vi "WinCI Add From SCC.vi"(8 "error in":errorcluster, 10 "files":path[](array[path]), 11 "source control reference in":T1) -> (0 "error out":errorcluster, 2 "status message":string, 3 "source control reference out":T1)   [LabVIEW 2017, in "NI_SCC_WinCI.lvlib"]
uses:
  <vilib>/SourceControl/Providers/WinCI/NI_SCC_WinCI.lvlib
  <vilib>/SourceControl/sccapi/SCCAPI Refnum.ctl
  <vilib>/SourceControl/sccapi/NI_SCC.lvlib
panel:
  out "result":i32
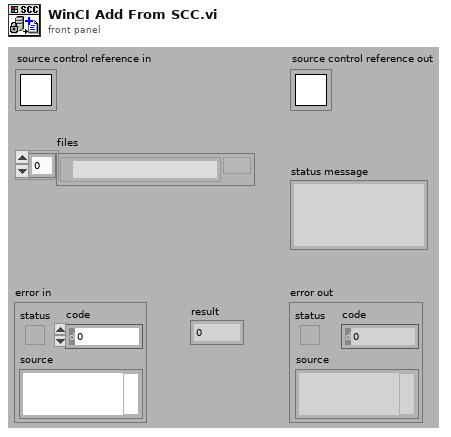
[diagram p1: front panel]
types:
  T1 = typedef "NI_SCC.lvlib/SCCAPI Refnum.ctl" = refnum<k1>
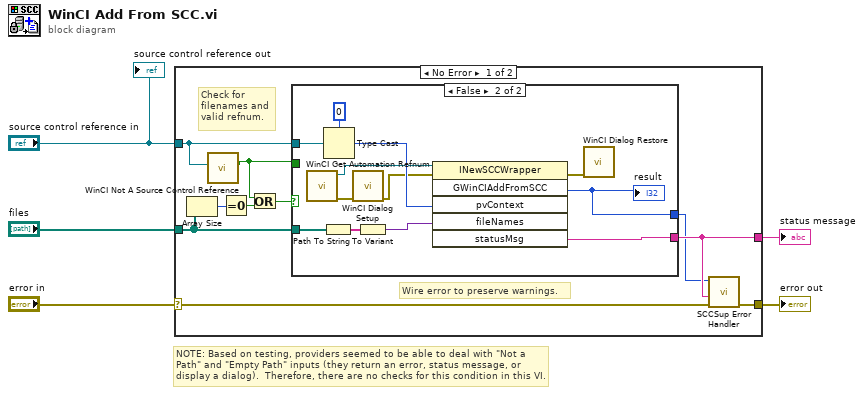
[diagram p0: block diagram]
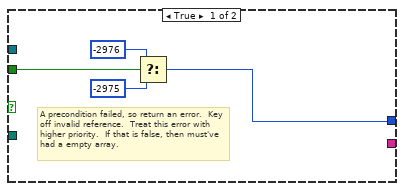
[diagram p2: hidden frame]
diagram:
  # "NOTE: Based on testing, providers seemed to be able to deal with \"Not a Path\" and \"Empty Path\" inputs (they return an error, status message, or display a dialog).  Therefore, there are no checks for this condition in this VI."
  n1 = case shown="No Error" "error in" {
    selector: "error in" -> [w8 w32]
    tunnel: [w14 w32] -> w4
    tunnel: "source control reference in" -> [w7 _]
    tunnel: [w13 _] -> w2
    tunnel: "files" -> [w15 _]
    frame No Error {
      # "Check for filenames and valid refnum."
      # "Wire error to preserve warnings."
      n2 = Array Size(array=w15) -> (size(s)=w10:i32)
      n3 = call <vilib>:"WinCI Not A Source Control Reference.vi"("source control reference in"=w7) -> ("not a source control reference?"=w6:bool)  [unwired: 1 in, 9 out]
      n4 = Equal To 0?(x=w10) -> (x = 0?=w11:bool)
      n5 = Or(x=w6, y=w11) -> (x .or. y?=w9:bool)
      n6 = case shown="False" w9 {
        tunnel: w7 -> [_ w31]
        tunnel: [_ w24] -> w13
        tunnel: w15 -> [_ w29]
        tunnel: [w16 w25] -> w12
        tunnel: w6 -> [w17 _]
        frame True {
          # "A precondition failed, so return an error.  Key off invalid reference.  Treat this error with higher priority.  If that is false, then must've had a empty array."
          n7 = Select(t=-2976 ("result"), s=w17, f=-2975 ("result")) -> (s? t:f=w16:i32)
        }
        frame False {
          n8 = call <vilib>:"WinCI Get Automation Refnum.vi"() -> ("error out"=w21:errorcluster, "automation refnum"=w22:refnum<k7>)  [unwired: 10 out]
          n9 = Path To String(path=w29) -> (string=w28:string[])
          n10 = Type Cast(type=u32 0, x=w31) -> (*(type *) &x=w26:u32)
          n11 = call <vilib>:"WinCI Dialog Setup.vi"("error in"=w21) -> ("error out"=w23:errorcluster)  [unwired: 10 out]
          n12 = To Variant(anything=w28) -> (Variant=w27:variant)
          n13 = invoke class="INewSCCWrapper" method="GWinCIAddFromSCC"(reference=w22, error in=w23, "pvContext"=w26, "fileNames"=w27) -> (error out=w20:errorcluster, "GWinCIAddFromSCC"=w25:i32, "statusMsg"=w24:string)  [unwired: 2 in, 3 out]
          "result" <- w25
          n14 = call <vilib>:"WinCI Dialog Restore.vi"("error in"=w20) -> ()  [unwired: 11 out]
        }
      }
      n15 = call <vilib>:"SCCSup Error Handler.vi"("error in (no error)"=w8, "additional message"=w13, "scc error code"=w12) -> ("error out"=w14:errorcluster)  [unwired: 1 in, 7 out]
    }
    frame Error {
    }
  }
  "error out" <- w4
  "status message" <- w2
  "source control reference out" <- "source control reference in"
